vi "ge_FileMods.vi"(5 "Config Grandmaster":T1) -> (2 "File Mods":string[](array[string]))   [LabVIEW 2011]
uses:
  Custom Ctrls/Master Cfg/ge_CfgGrandmaster.ctl
  Classes/GroupTiming/TimingGrp.lvclass
  Custom Ctrls/ge_ChassisType.ctl
  Custom Ctrls/ge_LockToLS.ctl
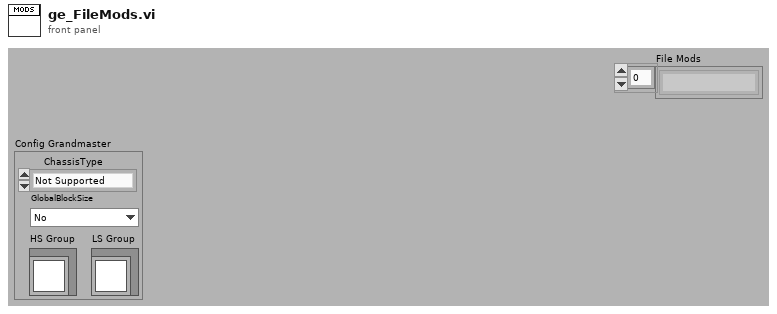
[diagram p1: front panel]
types:
  T1 = typedef "ge_CfgGrandmaster.ctl" = cluster{"ChassisType":T2, "GlobalBlockSize":T3, "HS Group":refnum<class "TimingGrp.lvclass">, "LS Group":refnum<class "TimingGrp.lvclass">}
  T2 = typedef "ge_ChassisType.ctl" = enum16{"Not Supported", "1-Slot", "4-Slot", "8-Slot"}
  T3 = typedef "ge_LockToLS.ctl" = enum16{"No", "250ms", "500ms", "1s"}
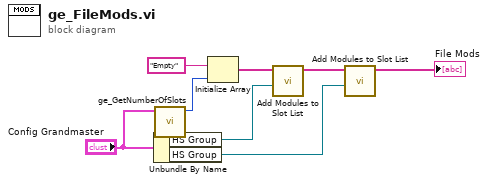
[diagram p0: block diagram]
diagram:
  n1 = Unbundle By Name("Config Grandmaster") -> ("HS Group"=w4:refnum<class "TimingGrp.lvclass">, "HS Group"=w2:refnum<class "TimingGrp.lvclass">)
  n2 = call "ge_GetNumberOfSlots.vi"("Config Grandmaster"="Config Grandmaster") -> ("# of Slots"=w6:i32)  [unwired: 10 in]
  n3 = Initialize Array("Empty", w6) -> (w5:string[])
  n4 = call "Add Modules to Slot List.vi"("TimingGrp in"=w4, "SlotMod List"=w5) -> ("Slot Mod Lilst"=w3:string[])  [unwired: 8 in, 1 out]
  n5 = call "Add Modules to Slot List.vi"("TimingGrp in"=w2, "SlotMod List"=w3) -> ("Slot Mod Lilst"=→"File Mods":string[])  [unwired: 8 in, 1 out]
